vi "Remove_end_return.vi"(1 "Input string":string) -> (0 "Output string":string)   [LabVIEW 2010]
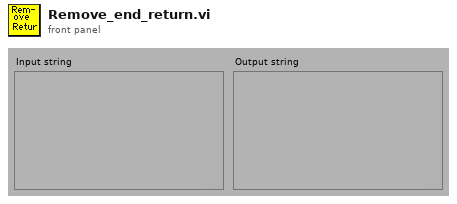
[diagram p1: front panel]
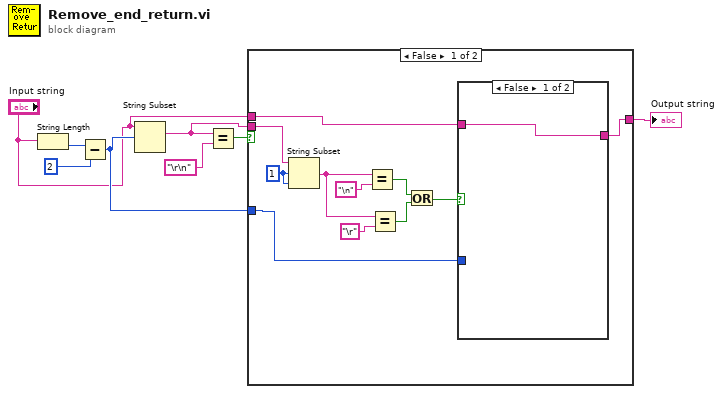
[diagram p0: block diagram]
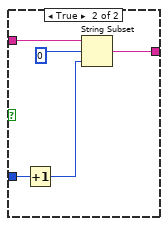
[diagram p2: hidden frame]
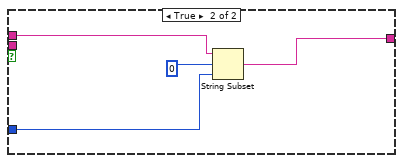
[diagram p3: hidden frame]
diagram:
  n1 = String Length(string="Input string") -> (length=w8:i32)
  n2 = Subtract(x=w8, y=2) -> (x-y=w4:i32)
  n3 = String Subset(string="Input string", offset (0)=w4) -> (substring=w1:string)  [unwired: 1 out]
  n4 = Equal?(x=w1, y="\r\n") -> (x = y?=w5:bool)
  n5 = case shown="False" w5 {
    tunnel: w4 -> [w10 w28]
    tunnel: "Input string" -> [w11 w27]
    tunnel: [w9 w26] -> w2
    tunnel: w1 -> [w18 _]
    frame False {
      w19 = 1 ("offset (0)")
      n6 = String Subset(string=w18, offset (0)=w19, length (rest)=w19) -> (substring=w15:string)
      n7 = Equal?(x=w15, y="\n") -> (x = y?=w13:bool)
      n8 = Equal?(x=w15, y="\r") -> (x = y?=w14:bool)
      n9 = Or(x=w13, y=w14) -> (x .or. y?=w12:bool)
      n10 = case shown="False" w12 {
        tunnel: w11 -> [w20 w24]
        tunnel: w10 -> [_ w23]
        tunnel: [w20 w21] -> w9
        frame False {
        }
        frame True {
          n11 = Increment(x=w23) -> (x+1=w22:i32)
          n12 = String Subset(string=w24, offset (0)=0, length (rest)=w22) -> (substring=w21:string)
        }
      }
    }
    frame True {
      n13 = String Subset(string=w27, offset (0)=0, length (rest)=w28) -> (substring=w26:string)
    }
  }
  "Output string" <- w2
